vi "Master Table Config File - Add Node.vi"(8 "error in (no error)":errorcluster, 10 "Local Channels Table Size In":u64, 11 "Compiled.Settings In":T1) -> (0 "error out":errorcluster, 3 "Compiled.Settings Out":T1)   [LabVIEW 2016, in "PXImc Custom Device System Explorer.lvlib"]
uses:
  PXImc Custom Device System Explorer.lvlib
  Shared/Compiled.Settings.ctl
  <vilib>/NI Veristand/VeriStand Data/Byte Buffer/Byte Buffer.lvclass
  PXImc Router/Controls/Target Type.ctl
  PXImc Router/Controls/Router - Configuration.ctl
  PXImc Router/Controls/Router/Node Block R-W Properties.ctl
  PXImc Router/Controls/Router/Block Properties.ctl
  PXImc Router/Controls/Router/Router - PXImc Properties.ctl
  PXImc Router/Controls/Router/Router - PXImc Card Properties.ctl
  PXImc Router/Controls/Node Data.ctl
  PXImc Router/Controls/Node/Node - PXImc Parameters.ctl
  PXImc Router/Controls/Node/Node - Writer Data.ctl
  PXImc Router/Controls/Node/Node Ch Properties.ctl
  PXImc Router/Controls/Data Type.ctl
  PXImc Router/Controls/Node/Node - Readers Data.ctl
  PXImc Router/Controls/Node/Node - Reader Data.ctl
  <vilib>/Utility/file.llb/Read Delimited Spreadsheet (string).vi
  <vilib>/Utility/file.llb/Write Delimited Spreadsheet (string).vi
  PXImc Router/PXImc Router.lvlib
  Shared/PXImc Custom Device Shared.lvlib
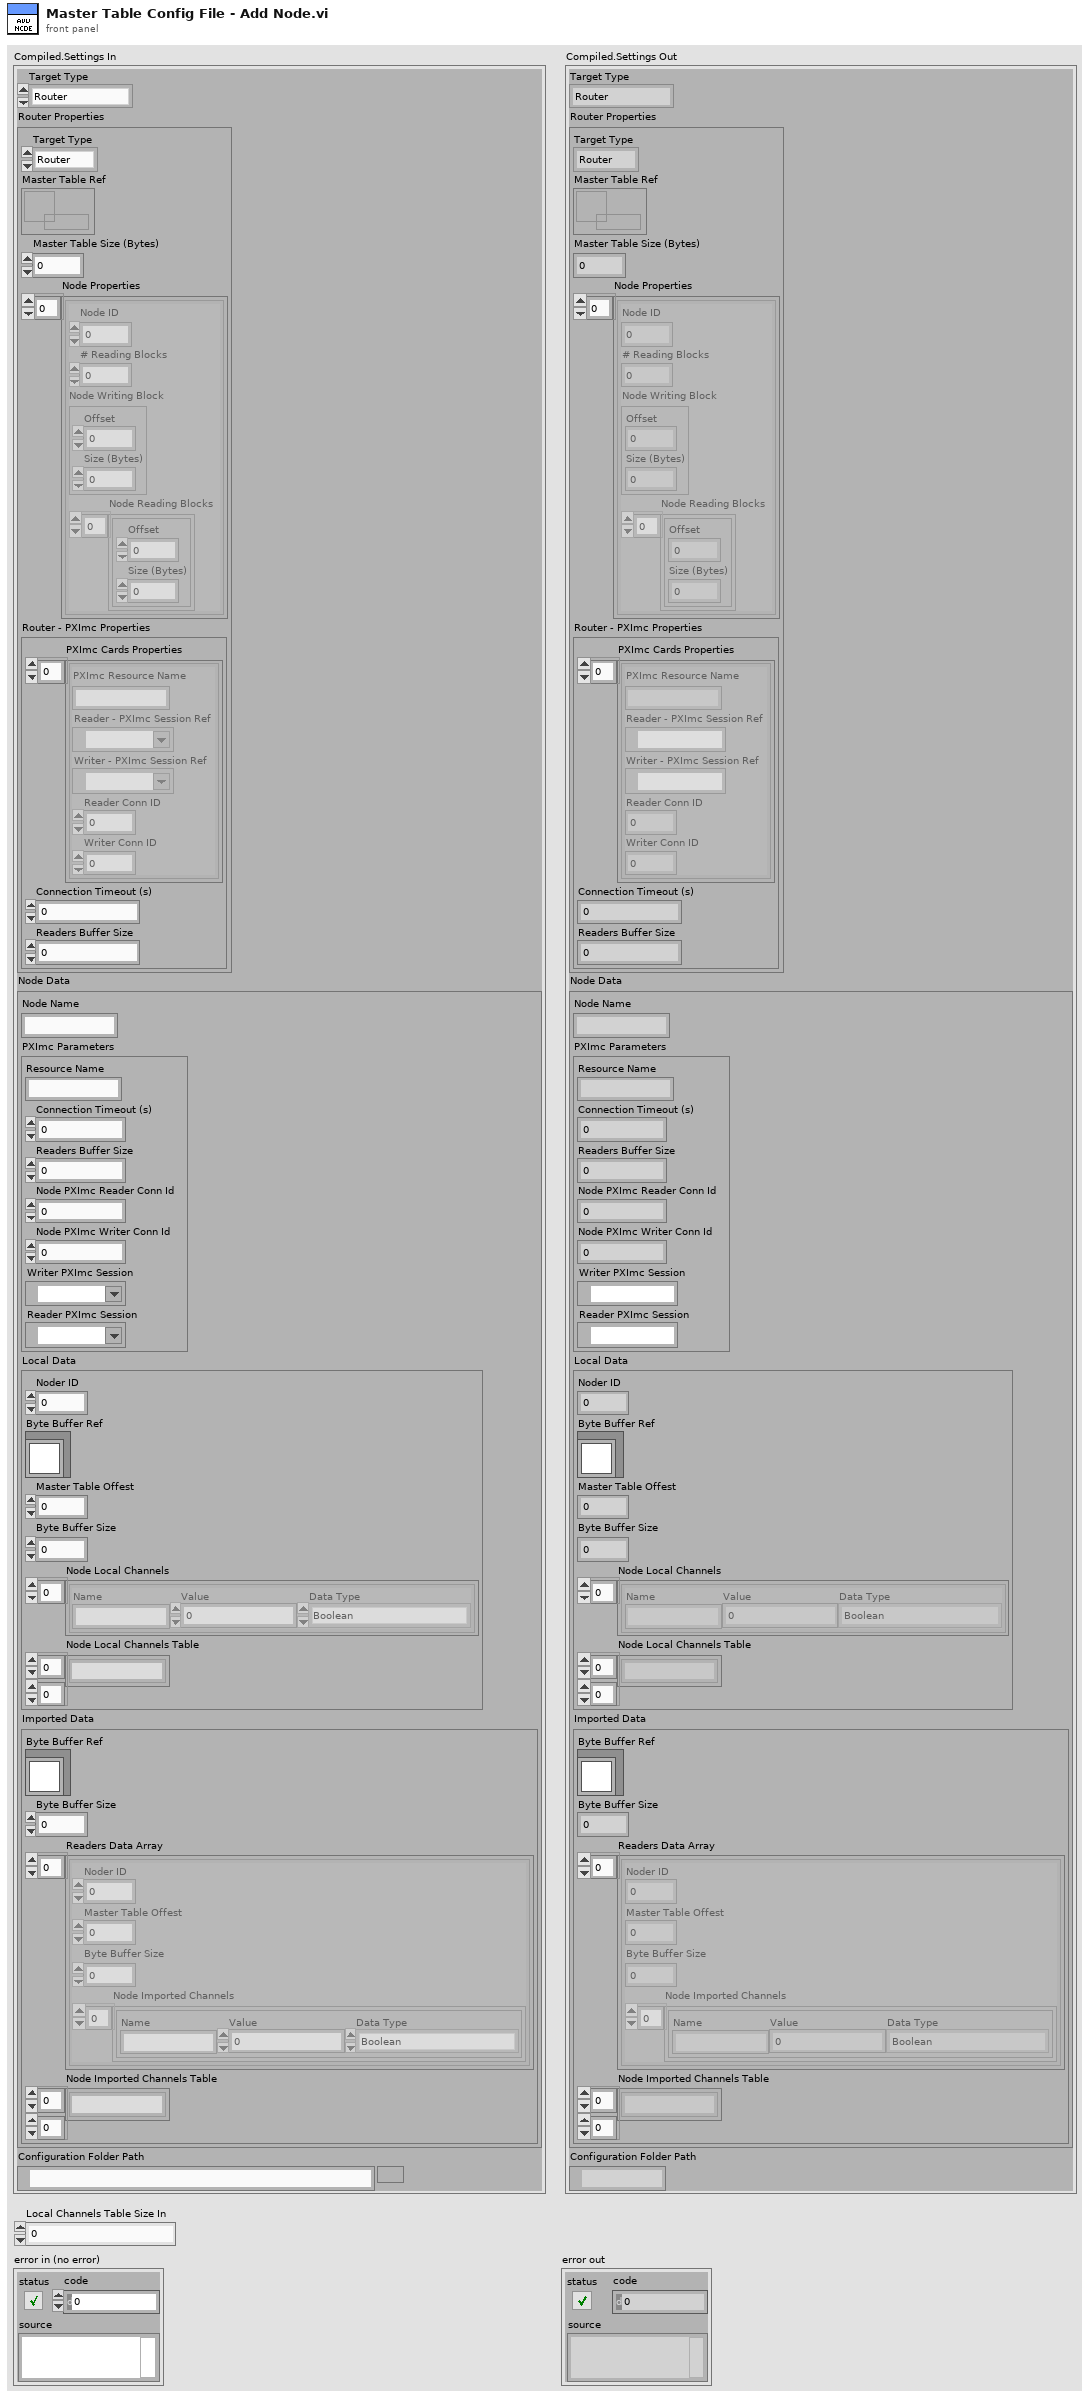
[diagram p1: front panel]
types:
  T1 = typedef "PXImc Custom Device Shared.lvlib/Compiled.Settings.ctl" = cluster{"Target Type":T2, "Router Properties":T3, "Node Data":T8, "Configuration Folder Path":path}
  T2 = typedef "PXImc Router.lvlib/Target Type.ctl" = enum16{"Router", "Node"}
  T3 = typedef "PXImc Router.lvlib/Router - Configuration.ctl" = cluster{"Target Type":T2, "Master Table Ref":refnum<data-value>, "Master Table Size (Bytes)":u32, "Node Properties":T4[], "Router - PXImc Properties":T6}
  T4 = typedef "PXImc Router.lvlib/Node Block R-W Properties.ctl" = cluster{"Node ID":u32, "# Reading Blocks":u32, "Node Writing Block":T5, "Node Reading Blocks":T5[]}
  T5 = typedef "PXImc Router.lvlib/Block Properties.ctl" = cluster{"Offset":u32, "Size (Bytes)":u32}
  T6 = typedef "PXImc Router.lvlib/Router - PXImc Properties.ctl" = cluster{"PXImc Cards Properties":T7[], "Connection Timeout (s)":dbl, "Readers Buffer Size":u64}
  T7 = typedef "PXImc Router.lvlib/Router - PXImc Card Properties.ctl" = cluster{"PXImc Resource Name":string, "Reader - PXImc Session Ref":refnum<k21>, "Writer - PXImc Session Ref":refnum<k21>, "Reader Conn ID":u16, "Writer Conn ID":u16}
  T8 = typedef "PXImc Router.lvlib/Node Data.ctl" = cluster{"Node Name":string, "PXImc Parameters":T9, "Local Data":T10, "Imported Data":T13}
  T9 = typedef "PXImc Router.lvlib/Node - PXImc Parameters.ctl" = cluster{"Resource Name":string, "Connection Timeout (s)":dbl, "Readers Buffer Size":u64, "Node PXImc Reader Conn Id":u16, "Node PXImc Writer Conn Id":u16, "Writer PXImc Session":refnum<k21>, "Reader PXImc Session":refnum<k21>}
  T10 = typedef "PXImc Router.lvlib/Node - Writer Data.ctl" = cluster{"Noder ID":u32, "Byte Buffer Ref":refnum<class "Byte Buffer.lvclass">, "Master Table Offest":u32, "Byte Buffer Size":u32, "Node Local Channels":T11[], "Node Local Channels Table":string[][]}
  T11 = typedef "PXImc Router.lvlib/Node Ch Properties.ctl" = cluster{"Name":string, "Value":dbl, "Data Type":T12}
  T12 = typedef "PXImc Router.lvlib/Data Type.ctl" = enum16{"Boolean", "SGL", "DBL", "I8", "I16", "I32", "I64", "U8", "U16", "U32", "U64"}
  T13 = typedef "PXImc Router.lvlib/Node - Readers Data.ctl" = cluster{"Byte Buffer Ref":refnum<class "Byte Buffer.lvclass">, "Byte Buffer Size":u64, "Readers Data Array":T14[], "Node Imported Channels Table":string[][]}
  T14 = typedef "PXImc Router.lvlib/Node - Reader Data.ctl" = cluster{"Noder ID":u32, "Master Table Offest":u32, "Byte Buffer Size":u64, "Node Imported Channels":T11[]}
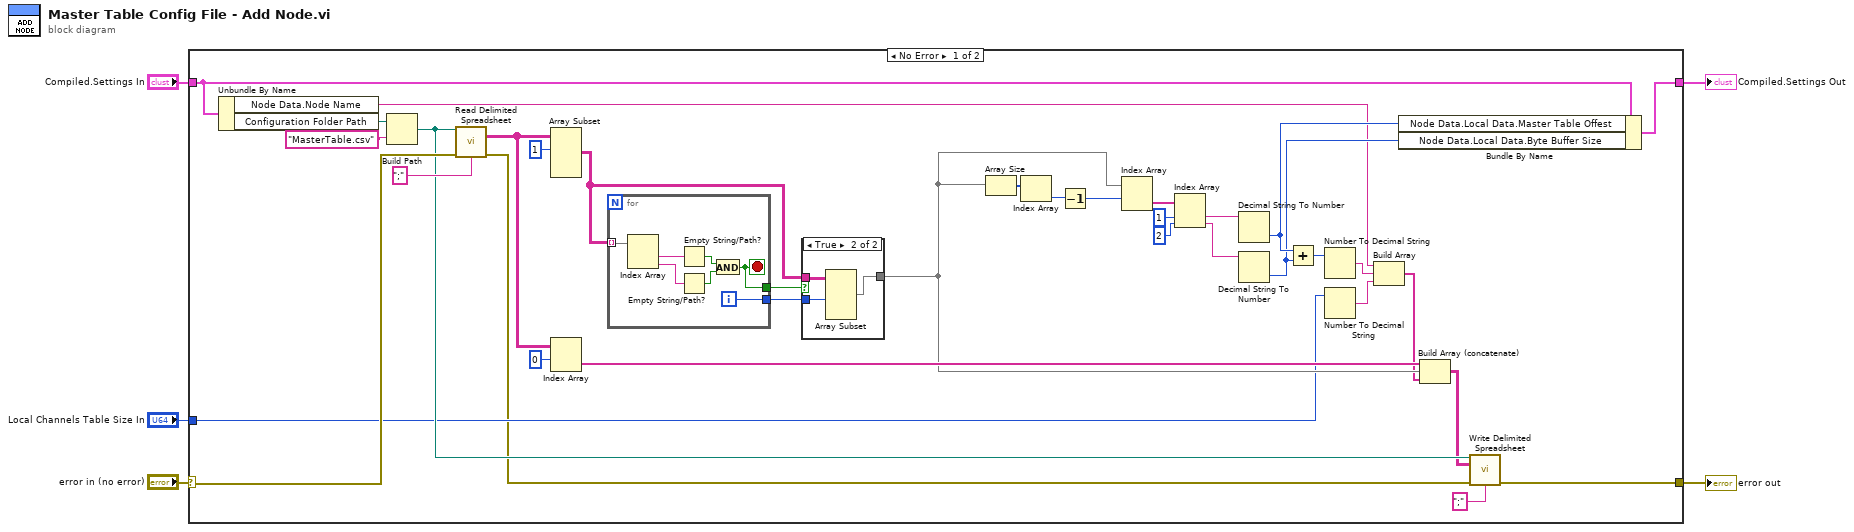
[diagram p0: block diagram]
diagram:
  n1 = case shown="No Error" "error in (no error)" {
    selector: "error in (no error)" -> [w39 w53]
    tunnel: [w9 w53] -> w4
    tunnel: "Compiled.Settings In" -> [w14 w52]
    tunnel: [w11 w52] -> w2
    tunnel: "Local Channels Table Size In" -> [w18 _]
    frame No Error {
      n2 = Unbundle By Name(w14) -> ("Node Data.Node Name"=w8:string, "Configuration Folder Path"=w38:path)
      n3 = Build Path(base path=w38, name or relative path="MasterTable.csv") -> (appended path=w26:path)
      n4 = call-poly <vilib>:"Read Delimited Spreadsheet.vi"("file path (dialog if empty)"=w26, "error in (no error)"=w39, "delimiter (\\t)"=";" ("delimiter (\\t)")) -> ("all rows"=w24:string[][], "error out"=w10:errorcluster)  [unwired: 7 in, 4 out]
      n5 = Array Subset(array=w24, index (row)=1 ("index")) -> (w29:string[][])  [unwired: 3 in]
      n6 = Index Array(array=w24, index (row)=0) -> (element=w22:string[])  [unwired: 1 in]
      n7 = for {
        tunnel: w29 -> [w49] mode=indexing
        tunnel: [w46] -> w27
        tunnel: [w45] -> w28
        i -> [w46]
        stop <- w45 stop-if-true
        n8 = Index Array(array=w49) -> (element #1=w50:string, element #2=w51:string)  [unwired: 2 in]
        n9 = Empty String/Path?(string/path=w50) -> (empty?=w48:bool)
        n10 = Empty String/Path?(string/path=w51) -> (empty?=w47:bool)
        n11 = And(x=w48, y=w47) -> (x .and. y?=w45:bool)
      }
      n12 = case shown="True" w28 {
        tunnel: [w41 w44] -> w21
        tunnel: w27 -> [_ w43]
        tunnel: w29 -> [w41 w42]
        frame False {
        }
        frame True {
          n13 = Array Subset(array=w42, length (row)=w43) -> (w44:string[][])  [unwired: 3 in]
        }
      }
      n14 = Array Size(array=w21) -> (size(s)=w35:i32[])
      n15 = Index Array(array=w35) -> (element=w33:i32)  [unwired: 1 in]
      n16 = Decrement(x=w33) -> (x-1=w34:i32)
      n17 = Index Array(array=w21, index (row)=w34) -> (element=w32:string[])  [unwired: 1 in]
      n18 = Index Array(array=w32, index #1=1 ("index"), index #2=2 ("index")) -> (element #1=w31:string, element #2=w30:string)
      n19 = Decimal String To Number(string=w31) -> (number=w13:i32)  [unwired: 2 in, 1 out]
      n20 = Decimal String To Number(string=w30) -> (number=w12:i32)  [unwired: 2 in, 1 out]
      n21 = Add(x=w13, y=w12) -> (x+y=w19:i32)
      n22 = Number To Decimal String(number=w19) -> (decimal integer string=w17:string)  [unwired: 1 in]
      n23 = Number To Decimal String(number=w18) -> (decimal integer string=w16:string)  [unwired: 1 in]
      n24 = Build Array(w8, w17, w16) -> (w15:string[])
      n25 = Bundle By Name(cluster=w14, "Node Data.Local Data.Master Table Offest"=w13, "Node Data.Local Data.Byte Buffer Size"=w12) -> (w11:T1)
      n26 = Build Array (concatenate)(w22, w21, w15) -> (w20:string[][])
      n27 = call-poly <vilib>:"Write Delimited Spreadsheet.vi"("file path (dialog if empty)"=w26, "2D data"=w20, "error in (no error)"=w10, "delimiter (\\t)"=";" ("delimiter (\\t)")) -> ("error out"=w9:errorcluster)  [unwired: 10 in, 1 out]
    }
    frame Error {
    }
  }
  "error out" <- w4
  "Compiled.Settings Out" <- w2
